vi "Add Observer.vi"(8 "error in (no error)":errorcluster, 10 "Observer":refnum<class "Observer.lvclass">, 11 "Observable in":refnum<class "Observable.lvclass">) -> (0 "error out":errorcluster, 3 "Observable out":refnum<class "Observable.lvclass">)   [LabVIEW 2011, in "Observable.lvclass"]
uses:
  Observable.lvclass
  Observer/Observer.lvclass
  Observable.lvclass/Observable.ctl
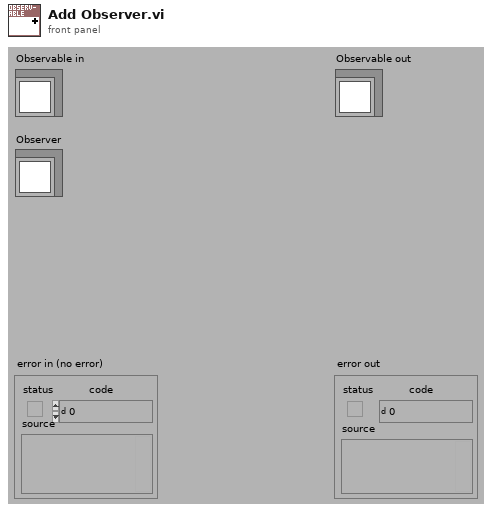
[diagram p1: front panel]
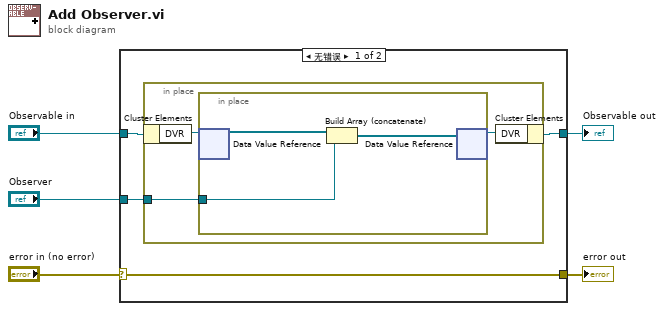
[diagram p0: block diagram]
diagram:
  n1 = case shown="无错误" "error in (no error)" {
    selector: "error in (no error)" -> [w6 w17]
    tunnel: "Observable in" -> [w9 w16]
    tunnel: [w8 w16] -> w4
    tunnel: "Observer" -> [w7 _]
    tunnel: [w6 w17] -> w1
    frame No Error {
      n2 = in-place {
        in-place-border: w7 -> [w10]
        n3 = in-place-cluster #1(w9) -> ("DVR"=w12:refnum<data-value>)
        n4 = in-place {
          in-place-border: w10 -> [w15]
          n5 = in-place-dvr #2(w12) -> (w14:refnum<class "Observer.lvclass">[])  [unwired: 1 out]
          n6 = Build Array (concatenate)(w14, w15) -> (w13:refnum<class "Observer.lvclass">[])
          n7 = in-place-dvr #2(w13) -> (w11:refnum<data-value>)  [unwired: 1 out]
        }
        n8 = in-place-cluster #1("DVR"=w11) -> (w8:refnum<class "Observable.lvclass">)
      }
    }
    frame Error {
    }
  }
  "Observable out" <- w4
  "error out" <- w1
